vi "OPV.vi"() -> ()   [LabVIEW 2017]
uses:
  EnumEstados1.ctl
  <vilib>/Analysis/3filter.llb/Filter Passband Type.ctl
  <vilib>/Analysis/NI_AALBase.lvlib
  <vilib>/Analysis/baseanly.llb/IIR Cascade Filter (DBL).vi
  <vilib>/Utility/NIReport.llb/NI_report.lvclass
  <vilib>/addons/_office/NI_ReportGenerationToolkit.lvlib
  <vilib>/addons/_office/excel.llb/Excel Easy Table (str).vi
panel:
  in  "Stop Button":bool
  in  "Save Button":bool
  in  "Guardar en:":path
  out "Voltage-Current Characterization:":cluster{dbl[], "Filtered X":dbl[]}(graph)
  in  "Ok":bool
  in  "order":i32=2
  in  "Numeric Control":dbl=0.01 format="%.2f"
  in  "Voltaje final:":dbl
  in  "Voltaje inicial:":dbl
  in  "Paso":dbl
  out "Eficiencia:":dbl
  out "Factor de Llenado:":dbl
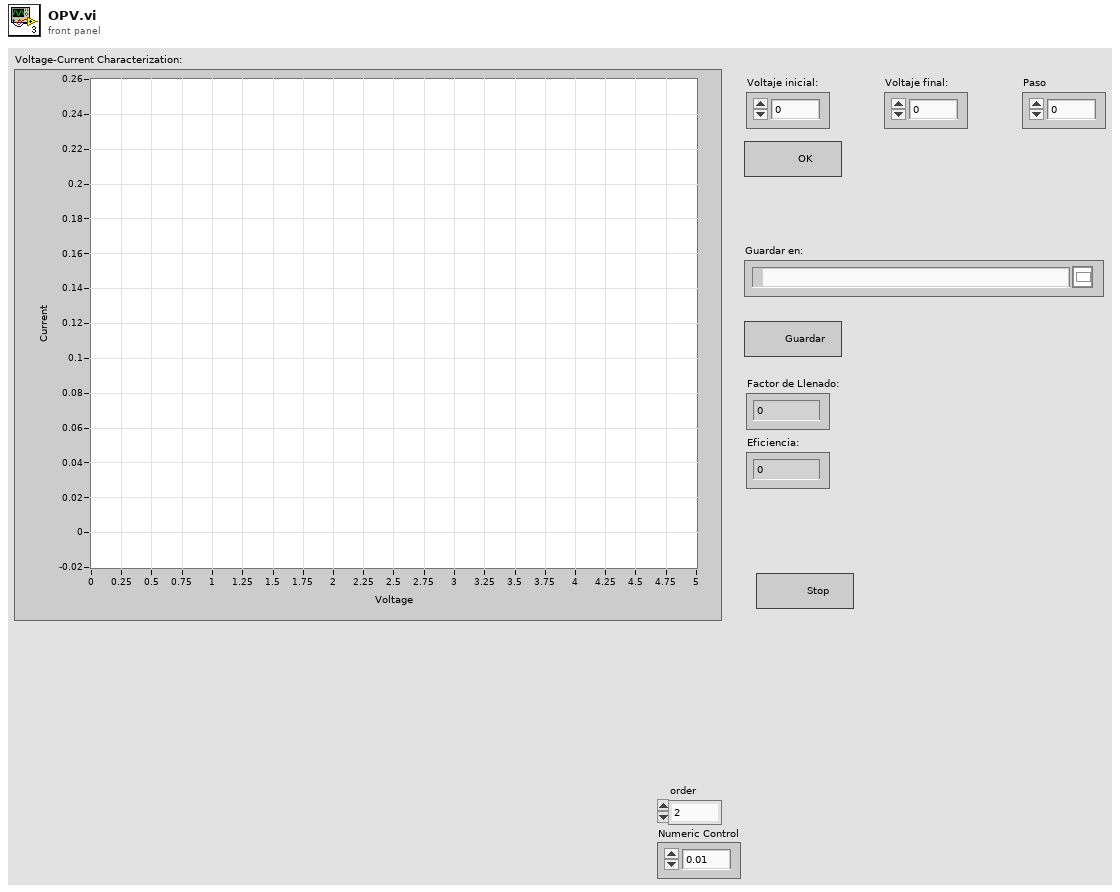
[diagram p1: front panel]
types:
  T1 = typedef "EnumEstados1.ctl" = enum16{"Inicio", "LecturaDatos", "Cierre"}
  T2 = typedef "NI_AALBase.lvlib/Filter Passband Type.ctl" = enum32{"Lowpass", "Highpass", "Bandpass", "Bandstop"}
  T3 = enum16{"Standard Report", "HTML", "Word", "Excel"}
  T4 = enum16{"maximized", "minimized", "normal", "no change"}
  T5 = enum16{"open", "open or create", "create or replace", "create", "open (read-only)"}
  T6 = cluster{"task out":refnum<k21>, "error out":errorcluster}
  T7 = cluster{"filter structure":enum32{"IIR 2nd Order", "IIR 4th Order"}, "Reverse Coefficients":dbl[], "Forward Coefficients":dbl[]}
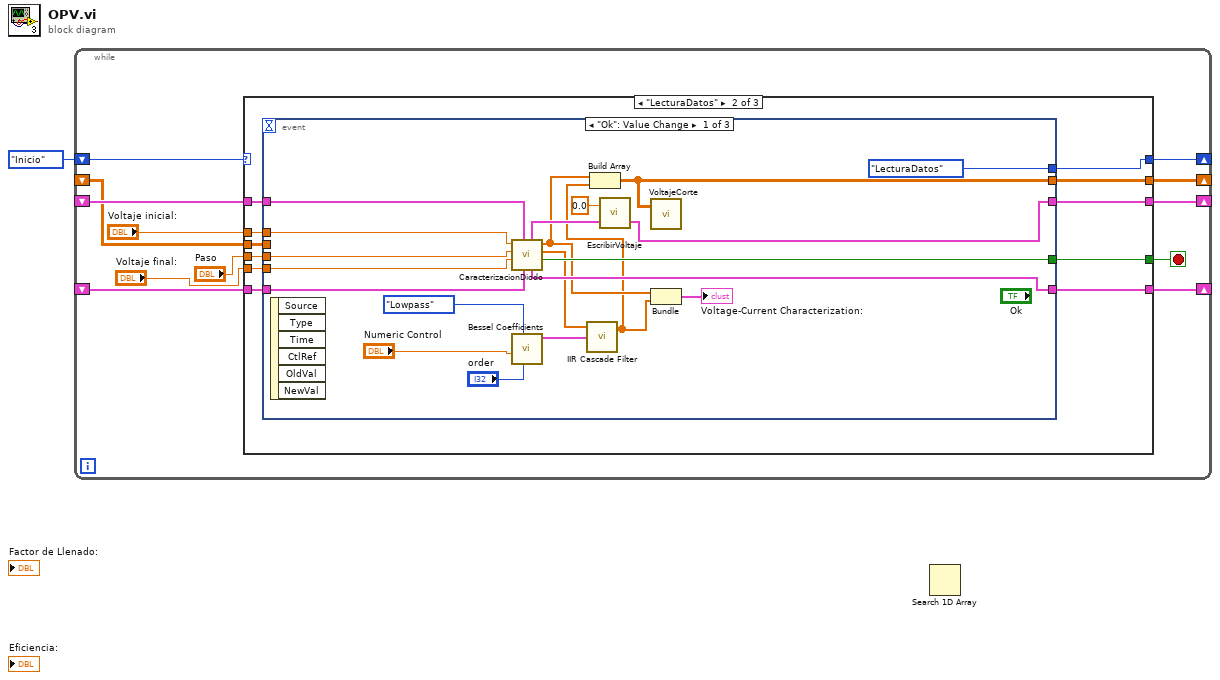
[diagram p0: block diagram]
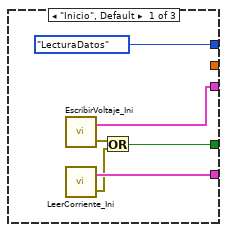
[diagram p2: hidden frame]
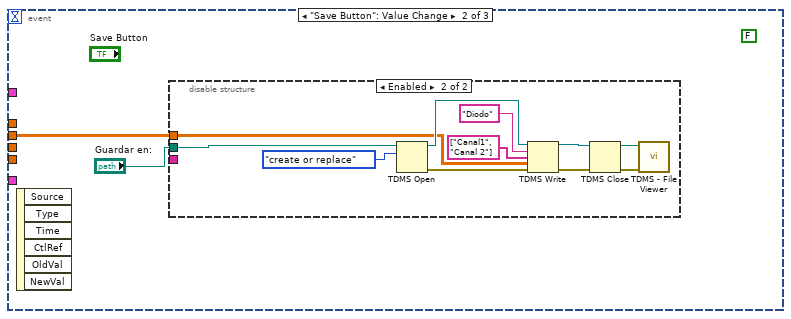
[diagram p3: hidden frame]
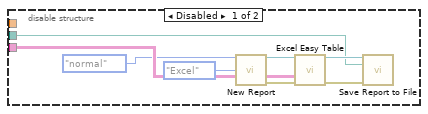
[diagram p4: hidden frame]
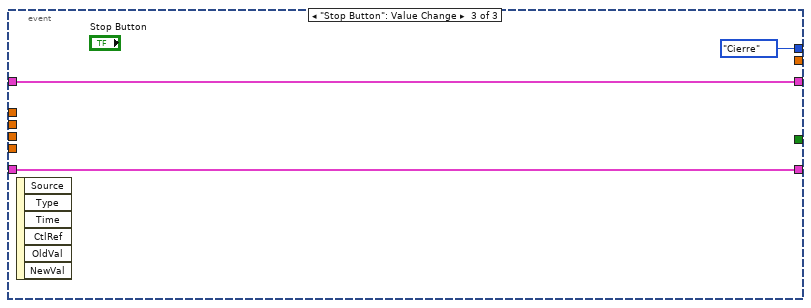
[diagram p5: hidden frame]
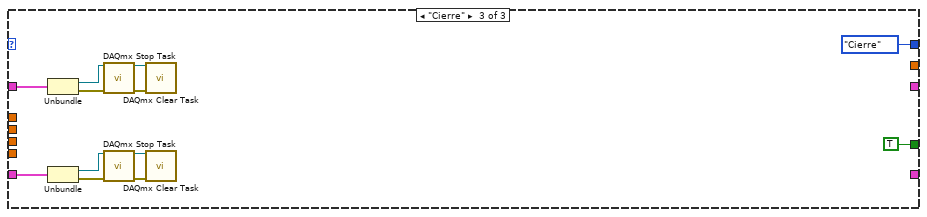
[diagram p6: hidden frame]
diagram:
  n1 = while {
    shift-right: [w5] -> _
    shift-left: EnumEstados1."Inicio" -> [w13]
    shift-right: [w9] -> _
    shift-left: _ -> [w8]
    shift-right: [w7] -> _
    shift-left: _ -> [w6]
    shift-right: [w4] -> _
    shift-left: _ -> [w3]
    stop <- w2 stop-if-true
    n2 = case shown="\"LecturaDatos\"" w13 {
      tunnel: "Voltaje final:" -> [_ w30 _]
      tunnel: "Voltaje inicial:" -> [_ w24 _]
      tunnel: "Paso" -> [_ w25 _]
      tunnel: [w18 w28 _] -> w9
      tunnel: w8 -> [_ w29 w82]
      tunnel: [w17 w26 _] -> w7
      tunnel: w6 -> [_ w27 w81]
      tunnel: [EnumEstados1."LecturaDatos" w23 EnumEstados1."Cierre"] -> w5
      tunnel: [_ w22 _] -> w4
      tunnel: w3 -> [_ w21 _]
      tunnel: [w14 w20 TRUE] -> w2
      frame "Inicio", Default {
        n3 = call "EscribirVoltaje_Ini.vi"() -> ("error out"=w16:errorcluster, "cluster"=w18:T6)  [unwired: 2 in]
        n4 = call "LeerCorriente_Ini.vi"() -> ("error out"=w15:errorcluster, "output cluster"=w17:T6)  [unwired: 2 in]
        n5 = Or(x=w16, y=w15) -> (x .or. y?=w14:bool)
      }
      frame "LecturaDatos" {
        n6 = event shown="[0] \"Ok\": Value Change" {
          selector: _ -> [_ _ _]
          dyn-events: _ -> [_ _ _]
          timeout: _ -> [_ _ _]
          tunnel: w30 -> [w41 _ _]
          tunnel: w29 -> [w40 _ w74]
          tunnel: [w46 _ w74] -> w28
          tunnel: w27 -> [w39 _ w73]
          tunnel: [w37 _ w73] -> w26
          tunnel: w25 -> [w42 _ _]
          tunnel: w24 -> [w43 _ _]
          tunnel: [EnumEstados1."LecturaDatos" _ EnumEstados1."Cierre"] -> w23
          tunnel: [w34 _ _] -> w22
          tunnel: w21 -> [_ w51 _]
          tunnel: [w35 _ _] -> w20
          event "Ok": Value Change {
            n7 = event-data() -> ()  [unwired: 1 in, 6 out]
            n8 = call "CaracterizacionDiodo.vi"("Corriente"=w39, "Voltaje"=w40, "Voltaje final:"=w41, "Paso"=w42, "Voltaje inicial:"=w43) -> ("Error?"=w35:bool, 2:"Corriente"=w33:dbl[], 3:"Voltaje"=w32:dbl[], 4:"Corriente"=w37:T6, 5:"Voltaje"=w38:T6)  [unwired: 2 in]
            n9 = call <vilib>:"Bessel Coefficients.vi"("order"="order", "filter type"=Filter_Passband_Type."Lowpass", "low cutoff freq: fl"="Numeric Control") -> ("IIR Filter Cluster"=w49:T7)  [unwired: 7 in, 1 out]
            n10 = call-poly <vilib>:"IIR Cascade Filter.vi"("IIR Filter Cluster"=w49, "X"=w33) -> ("Filtered X"=w31:dbl[])  [unwired: 1 in, 1 out]
            n11 = Build Array(w32, w31) -> (w34:dbl[][])
            n12 = call "EscribirVoltaje.vi"("cluster"=w38, "data"=0.0) -> ("Cluster"=w46:T6)  [unwired: 1 out]
            n13 = call "VoltajeCorte.vi"("Array in"=w34) -> ()  [unwired: 1 in, 2 out]
            n14 = Bundle("Voltaje"=w32, "Filtered X"=w31) -> (→"Voltage-Current Characterization:":cluster{"Voltaje":dbl[], "Filtered X":dbl[]})  [unwired: 1 in]
          }
          event "Save Button": Value Change {
            (unwired) FALSE
            n15 = event-data() -> ()  [unwired: 1 in, 6 out]
            n16 = disable-structure shown="Enabled" {
              disable-tunnel: _ -> [w58 _]
              disable-tunnel: "Guardar en:" -> [w53 w64]
              disable-tunnel: w51 -> [_ w61]
              frame Disabled {
                n17 = call <vilib>:"New Report.vi"("window state (normal)"=T4."normal", "report type"=T3."Excel") -> ("report out"=w60:refnum<class "NI_report.lvclass">, "error out"=w59:errorcluster)  [unwired: 12 in]
                n18 = call-poly <vilib>:"Excel Easy Table.vi"("report in"=w60, "text data"=w58, "error in (no error)"=w59) -> ("report out"=w57:refnum<class "NI_report.lvclass">, "error out"=w56:errorcluster)  [unwired: 8 in, 3 out]
                n19 = call-dynamic "Save Report to File.vi"("report in"=w57, "report file path"=w53, "error in (no error)"=w56) -> ()  [unwired: 11 in, 2 out]
              }
              frame Enabled {
                n20 = TDMS Open(10:T5."create or replace" ("operation (0:open)"), 11:w64) -> (0:w68:errorcluster, 3:w65:refnum<k34>)  [unwired: 5 in]
                n21 = TDMS Write(0:w65, 5:"Diodo" ("group name in (Untitled)"), 7:string[] ["Canal1", "Canal 2"] ("channel name(s) in (Untitled)"), 9:w61, 11:w68) -> (4:w66:refnum<k34>, 15:w67:errorcluster)  [unwired: 1 in, 2 out]
                n22 = TDMS Close(8:w67, 11:w66) -> (0:w63:errorcluster, 3:w62:path)
                n23 = call <vilib>:"TDMS - File Viewer.vi"("error in (no error)"=w63, "file path"=w62) -> ()  [unwired: 4 in, 2 out]
              }
            }
          }
          event "Stop Button": Value Change {
            n24 = event-data() -> ()  [unwired: 1 in, 6 out]
          }
        }
      }
      frame "Cierre" {
        n25 = Unbundle(w82) -> ("task out"=w80:refnum<k21>, "error out"=w79:errorcluster)
        n26 = Unbundle(w81) -> ("task out"=w78:refnum<k21>, "error out"=w77:errorcluster)
        n27 = call <vilib>:"DAQmx Stop Task.vi"("task/channels in"=w80, "error in"=w79) -> ("task out"=w86:refnum<k21>, "error out"=w85:errorcluster)  [unwired: 12 in]
        n28 = call <vilib>:"DAQmx Stop Task.vi"("task/channels in"=w78, "error in"=w77) -> ("task out"=w84:refnum<k21>, "error out"=w83:errorcluster)  [unwired: 12 in]
        n29 = call <vilib>:"DAQmx Clear Task.vi"("task in"=w86, "error in"=w85) -> ()  [unwired: 13 in, 1 out]
        n30 = call <vilib>:"DAQmx Clear Task.vi"("task in"=w84, "error in"=w83) -> ()  [unwired: 13 in, 1 out]
      }
    }
  }
  n31 = Search 1D Array() -> ()  [unwired: 3 in, 1 out]
